vi "Read Current Position.vi"(8 "error in (no error)":errorcluster, 11 "Sync 2-Axis Stage Controller in":refnum<class "Sync 2-Axis Stage Controller.lvclass">) -> (0 "error out":errorcluster, 1 "Y Position":dbl, 2 "X Position":dbl, 3 "Sync 2-Axis Stage Controller out":refnum<class "Sync 2-Axis Stage Controller.lvclass">)   [LabVIEW 2022 SP3, in "Sync 2-Axis Stage Controller.lvclass"]
uses:
  Sync 2-Axis Stage Controller.lvclass
  Sync 2-Axis Stage Controller.lvclass/Sync 2-Axis Stage Controller.ctl
  Axis Objects/iMotion Controller/iMotion Controller.lvclass
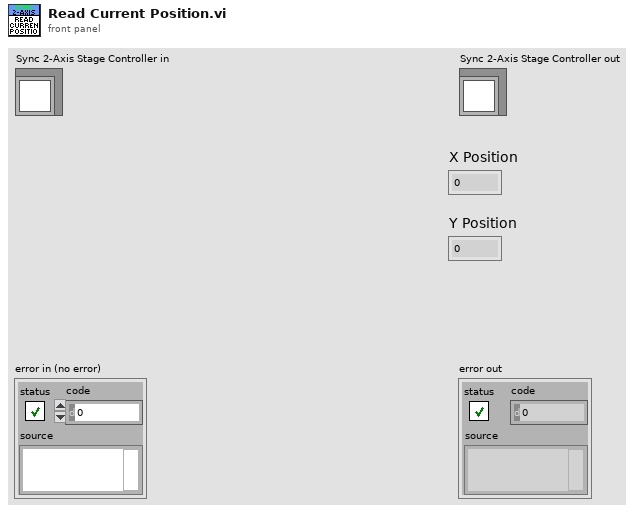
[diagram p1: front panel]
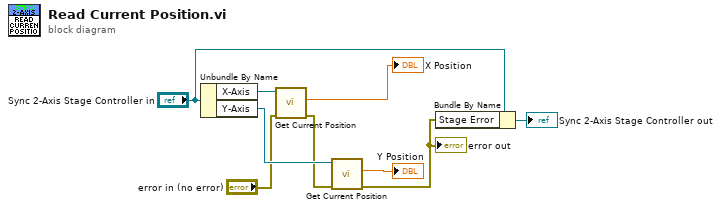
[diagram p0: block diagram]
diagram:
  n1 = Unbundle By Name("Sync 2-Axis Stage Controller in") -> ("X-Axis"=w8:refnum<class "iMotion Controller.lvclass">, "Y-Axis"=w7:refnum<class "iMotion Controller.lvclass">)
  n2 = call-dynamic "Get Current Position.vi"("error in (no error)"="error in (no error)", "iMotion Controller in"=w8) -> ("error out"=w1:errorcluster, "Current Position"=→"X Position":dbl)  [unwired: 7 in, 1 out]
  n3 = call-dynamic "Get Current Position.vi"("error in (no error)"=w1, "iMotion Controller in"=w7) -> ("error out"=w6:errorcluster, "Current Position"=→"Y Position":dbl)  [unwired: 7 in, 1 out]
  "error out" <- w6
  n4 = Bundle By Name(cluster="Sync 2-Axis Stage Controller in", "Stage Error"=w6) -> (→"Sync 2-Axis Stage Controller out":refnum<class "Sync 2-Axis Stage Controller.lvclass">)
